vi "Decel.vi"(6 "EncData":T1) -> (3 "SpdMult":dbl)   [LabVIEW 2017]
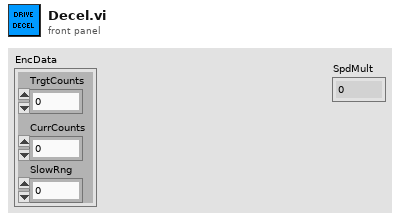
[diagram p1: front panel]
types:
  T1 = cluster{"TrgtCounts":i32, "CurrCounts":dbl, "SlowRng":dbl}
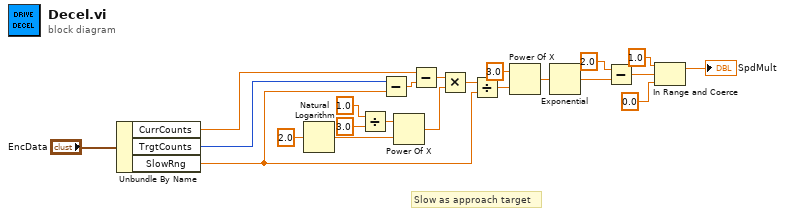
[diagram p0: block diagram]
diagram:
  # "Slow as approach target"
  n1 = Unbundle By Name("EncData") -> ("CurrCounts"=w5:dbl, "TrgtCounts"=w6:i32, "SlowRng"=w2:dbl)
  n2 = Natural Logarithm(1:2.0 ("x")) -> (0:w12:dbl)
  n3 = Divide(x=1.0, y=3.0 ("x")) -> (x/y=w13:dbl)
  n4 = Subtract(x=w6, y=w2) -> (x-y=w9:dbl)
  n5 = Power Of X(1:w12, 2:w13) -> (0:w16:dbl)
  n6 = Subtract(x=w5, y=w9) -> (x-y=w10:dbl)
  n7 = Multiply(x=w10, y=w16) -> (x*y=w17:dbl)
  n8 = Divide(x=w17, y=w2) -> (x/y=w18:dbl)
  n9 = Power Of X(1:w18, 2:3.0 ("x")) -> (0:w20:dbl)
  n10 = Exponential(1:w20) -> (0:w21:dbl)
  n11 = Subtract(x=2.0, y=w21) -> (x-y=w8:dbl)
  n12 = In Range and Coerce(upper limit=1.0 ("f"), x=w8, lower limit=0.0) -> (coerced(x)=→"SpdMult":dbl)  [unwired: 1 out]
